vi "Update Value.vi"(6 "Time":dbl, 8 "error in (no error)":errorcluster, 11 "GuiLinkButton in":refnum<class "GuiLinkButton.lvclass">) -> (0 "error out":errorcluster, 1 "Update":bool, 2 "Value":variant, 3 "GuiLinkButton out":refnum<class "GuiLinkButton.lvclass">)   [LabVIEW 2020, in "VolatusGUIElements.lvlib" / "GuiLinkButton.lvclass"]
uses:
  GuiLinkButton.lvclass
  GuiLinkButton.lvclass/GuiLinkButton.ctl
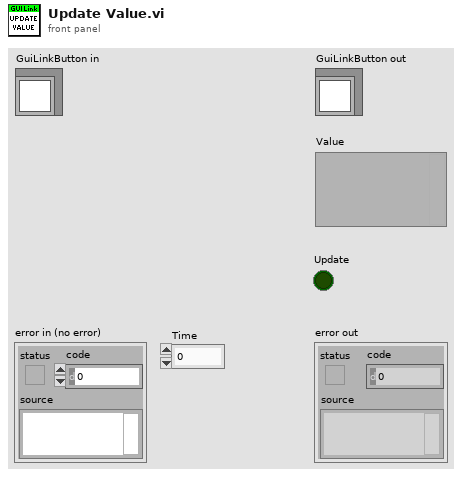
[diagram p1: front panel]
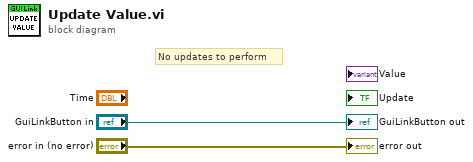
[diagram p0: block diagram]
diagram:
  # "No updates to perform"
  "error out" <- "error in (no error)"
  "GuiLinkButton out" <- "GuiLinkButton in"
